vi "Sub Super Duper_6_14b_JW.vi"(0 "VISA resource name":refnum<visa-resource-name>="GPIB0::17::INSTR", 1 "Sample Properties:":T5 {"Date Created" format="%<%Y/%m/%d>T"}, 2 "TRF Cluster":T6={"Step 4"=-38.0, "# of Loops"=1.0, "Transfer 2"=FALSE, "Start 4"=-2.0, "Total Points 2"=2, "Start 3"=40.0, "Stop 2"=-40.0, "Step 3"=-1.0, "Loop Step"=0.0, "Integration Time 3"=0, "Loop Wait"=0.0, "First Step"=0.0} {"Loop Wait" format="%<%H:%M:%S>t"; "Integration Time 3" scale=0.0..2.0; "Step 3" format="%.2f"; "Stop 2" format="%.2f"; "Start 3" format="%.2f"; "Start 4" format="%.2f"; "Step 4" format="%.2f"}, 3 "TSP Cluster":T7={"Transport"=FALSE, "Start 2"=0.0, "Stop 3"=-60.0, "Step 2"=-1.0, "Start"=0.0, "Step"=-10.0, "Total Points"=7, "Integration Time"=0} {"Integration Time" scale=0.0..2.0; "Step" format="%.2f"; "Start" format="%.2f"; "Step 2" format="%.2f"; "Stop 3" format="%.2f"; "Start 2" format="%.2f"}, 4 "Compliance Cluster":T2={"Var1 sweep settings"={"sweep spacing (linear: 0)"=0, "sweep mode"=FALSE, "compliance (V)"=100.0, "compliance (A)"=0.001}, "Var1 sweep settings 2"={"sweep spacing (linear: 0)"=0, "sweep mode"=FALSE, "compliance (V)"=100.0, "compliance (A)"=0.001}, "Var2 step settings 2"={"compliance (A)"=0.001, "compliance (V)"=100.0}, "Var2 step settings"={"compliance (A)"=0.001, "compliance (V)"=100.0}} {"Var2 step settings"."compliance (V)" format="%.2f"; "Var2 step settings"."compliance (A)" format="%^.2e"; "Var2 step settings 2"."compliance (V)" format="%.2f"; "Var2 step settings 2"."compliance (A)" format="%^.2e"; "Var1 sweep settings 2"."compliance (A)" format="%^.2e"; "Var1 sweep settings 2"."compliance (V)" format="%.2f"; "Var1 sweep settings 2"."sweep spacing (linear: 0)" items=["linear", "log 10", "log 25", "log 50"]; "Var1 sweep settings"."compliance (A)" format="%^.2e"; "Var1 sweep settings"."compliance (V)" format="%.2f"; "Var1 sweep settings"."sweep spacing (linear: 0)" items=["linear", "log 10", "log 25", "log 50"]}, 5 "error in":errorcluster, 6 "Saved Folder:":path=path "C:/1DATA/2011", 7 "Wait Cluster":T1 {"Wait Time (s)" format="%.1g"; "Wait Countdown" format="%<%H:%M:%S%1u>t"}, 9 "Stop \nCountdown":bool) -> (8 "Status Indicator":bool, 14 "VISA resource name out":refnum<visa-resource-name>, 15 "TRF Path":path, 16 "TSP Path":path, 17 "Graph Cluster":T3, 18 "Char Cluster":T4, 19 "error out":errorcluster)   [LabVIEW 2011]
uses:
  <vilib>/Platform/TimedLoop/XDataNode/timing_clust.ctl
  <vilib>/Platform/TimedLoop/XDataNode/nitl_modes.ctl
  <vilib>/Platform/TimedLoop/XDataNode/wakeup.ctl
  <vilib>/Platform/TimedLoop/XDataNode/XDataNode.xnode
  <vilib>/Platform/TimedLoop/XDataNode/XDNodeRunTimeDep.lvlib
panel:
  in  "Transport Temp":cluster{"trace":dbl[], "trace":dbl[]}(graph)
  in  "Transfer Temp":cluster{dbl[], "trace":dbl[]}[](graph) caption="Transfer"
  out "graphic display":cluster{"trace":dbl[], "trace":dbl[]}(graph)
  # "Vg Sweep"
  # "Vd Step"
  # "Loops and Integration Time"
  # "Device Characteristics"
  # "Sample Properties:"
  # "%"
  # "nm"
  # "Device Properties:"
  # "um"
  # "um"
  # "Vg Step"
  # "Vd Step"
  # "Integration Time"
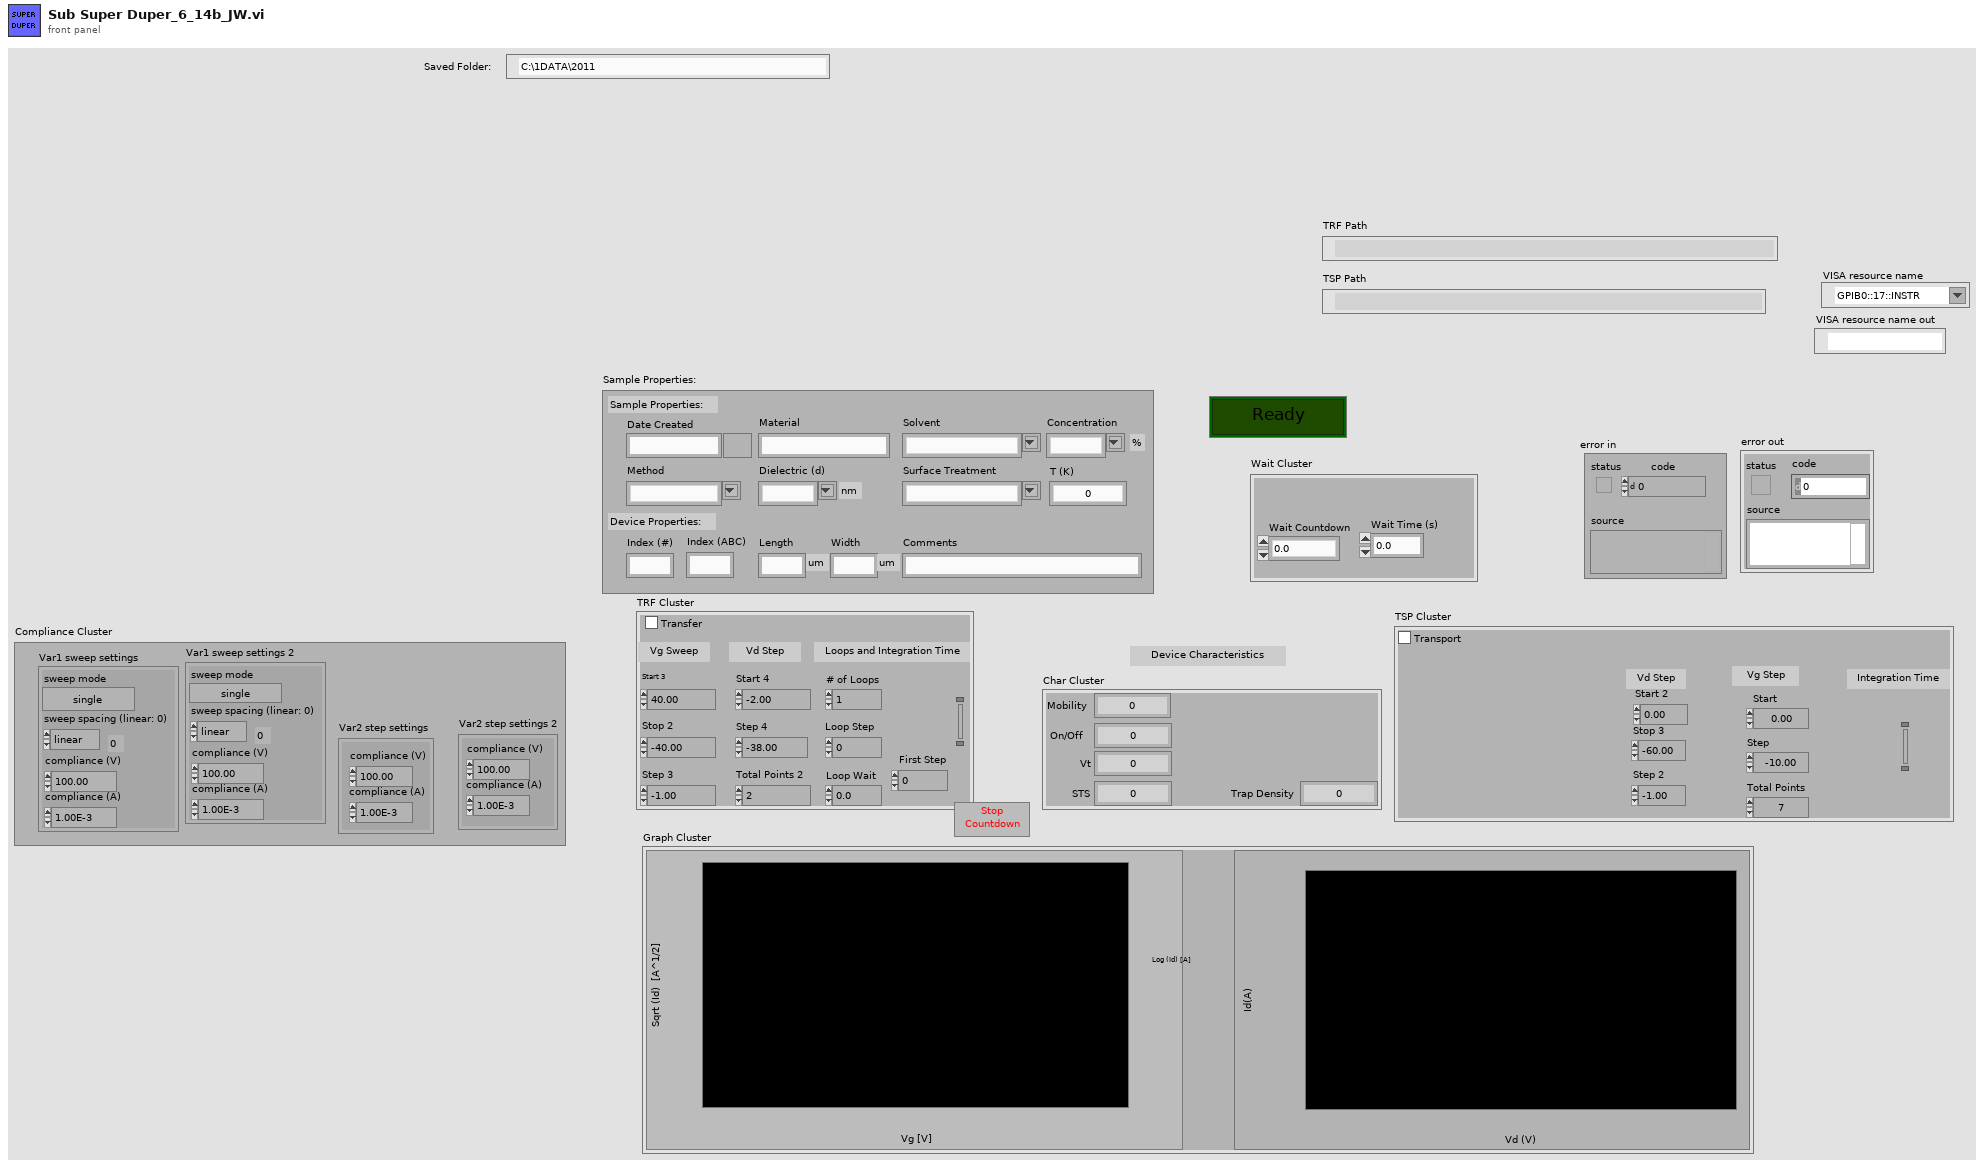
[diagram p1: front panel]
types:
  T1 = cluster{"Wait Countdown":dbl, "Wait Time (s)":dbl}
  T2 = cluster{"Var1 sweep settings":cluster{"sweep spacing (linear: 0)":u16, "sweep mode":bool, "compliance (V)":dbl, "compliance (A)":dbl}, "Var1 sweep settings 2":cluster{"sweep spacing (linear: 0)":u16, "sweep mode":bool, "compliance (V)":dbl, "compliance (A)":dbl}, "Var2 step settings 2":cluster{"compliance (A)":dbl, "compliance (V)":dbl}, "Var2 step settings":cluster{"compliance (A)":dbl, "compliance (V)":dbl}}
  T3 = cluster{"Transfer":cluster{dbl[], "trace":dbl[]}[], "Transport":cluster{"trace":dbl[], "trace":dbl[]}}
  T4 = cluster{"Mobility":dbl, "On/Off ":dbl, "Vt":dbl, "STS":dbl, "Trap Density":dbl}
  T5 = cluster{"Date Created":timestamp, "Material":string, "Solvent":string, "Concentration":string, "Method":string, "Dielectric (d)":string, "Index (#)":string, "Index (ABC)":string, "Length":string, "Width":string, "Surface Treatment":string, "Comments":string, "T (K)":dbl}
  T6 = cluster{"Step 4":dbl, "# of Loops":dbl, "Transfer 2":bool, "Start 4":dbl, "Total Points 2":u16, "Start 3":dbl, "Stop 2":dbl, "Step 3":dbl, "Loop Step":dbl, "Integration Time 3":u32, "Loop Wait":dbl, "First Step":dbl}
  T7 = cluster{"Transport":bool, "Start 2":dbl, "Stop 3":dbl, "Step 2":dbl, "Start":dbl, "Step":dbl, "Total Points":u16, "Integration Time":u32}
  T8 = typedef "XDNodeRunTimeDep.lvlib/timing_clust.ctl" = cluster{"Expected End [f-1]":u64, "Actual End [f-1]":u64, "Finished Late? [f-1]":bool, "Expected End [i-1]":u64, "Actual End [i-1]":u64, "Finished Late? [i-1]":bool, "Expected Start [i]":u64, "Actual Start [i]":u64, "Expected Start [f]":u64, "Actual Start [f]":u64, "Source Name":string, "Structure Name":string, "Period":i64, "Deadline":i64, "Offset":i64, "Start":i64, "Priority":i32, "Timeout":i32, "Mode":T9, "Wakeup Reason":T10, "Error":errorcluster, "Source Type":string, "Secondary Source Type":string, "Global End Time":u64, "Global Start Time":u64, "Frame Duration":u64, "Iteration Duration":u64, "Assigned CPU":i32, "I/O Scan Engine Mode":u32}
  T9 = typedef "XDNodeRunTimeDep.lvlib/nitl_modes.ctl" = enum32{"No Change", "Process missed periods, maintain original phase", "Discard missed periods, maintain original phase", "Process missed periods, ignore original phase", "Discard missed periods, ignore original phase"}
  T10 = typedef "XDNodeRunTimeDep.lvlib/wakeup.ctl" = enum32{"Normal", "Aborted", "Asynchronous wakeup", "Timing source error", "Timed loop error", "Timeout"}
  T11 = cluster{"sweep spacing (linear: 0)":u16, "sweep mode":bool, "compliance (V)":dbl, "compliance (A)":dbl}
  T12 = cluster{"compliance (A)":dbl, "compliance (V)":dbl}
  T13 = cluster{"Start 3":dbl, "Stop 2":dbl, "Step 3":dbl, "sweep spacing (linear: 0)":u16, "sweep mode":bool, "compliance (V)":dbl, "compliance (A)":dbl}
  T14 = cluster{"compliance (A)":dbl, "compliance (V)":dbl, "Start 4":dbl, "Total Points 2":u16, dbl}
  T15 = cluster{"Step 4":dbl, "# of Loops":dbl, "Transfer 2":bool, "Start 4":dbl, "Total Points 2":u16, "Start 3":dbl, "Stop 2":dbl, "Step 3":dbl, dbl, "Integration Time 3":u32, "Loop Wait":dbl, "First Step":dbl}
  T16 = cluster{"Mobility":dbl, "On/Off Current":dbl, "Vt":dbl, "Trap Density":dbl, "STS":dbl}
  T17 = cluster{"Start 2":dbl, "Stop 3":dbl, "Step 2":dbl, "sweep spacing (linear: 0)":u16, "sweep mode":bool, "compliance (V)":dbl, "compliance (A)":dbl}
  T18 = cluster{"compliance (A)":dbl, "compliance (V)":dbl, "Start":dbl, "Total Points":u16, "Step":dbl}
  T19 = cluster{"Transfer Temp":cluster{dbl[], "trace":dbl[]}[], "Transport Temp":cluster{"trace":dbl[], "trace":dbl[]}}
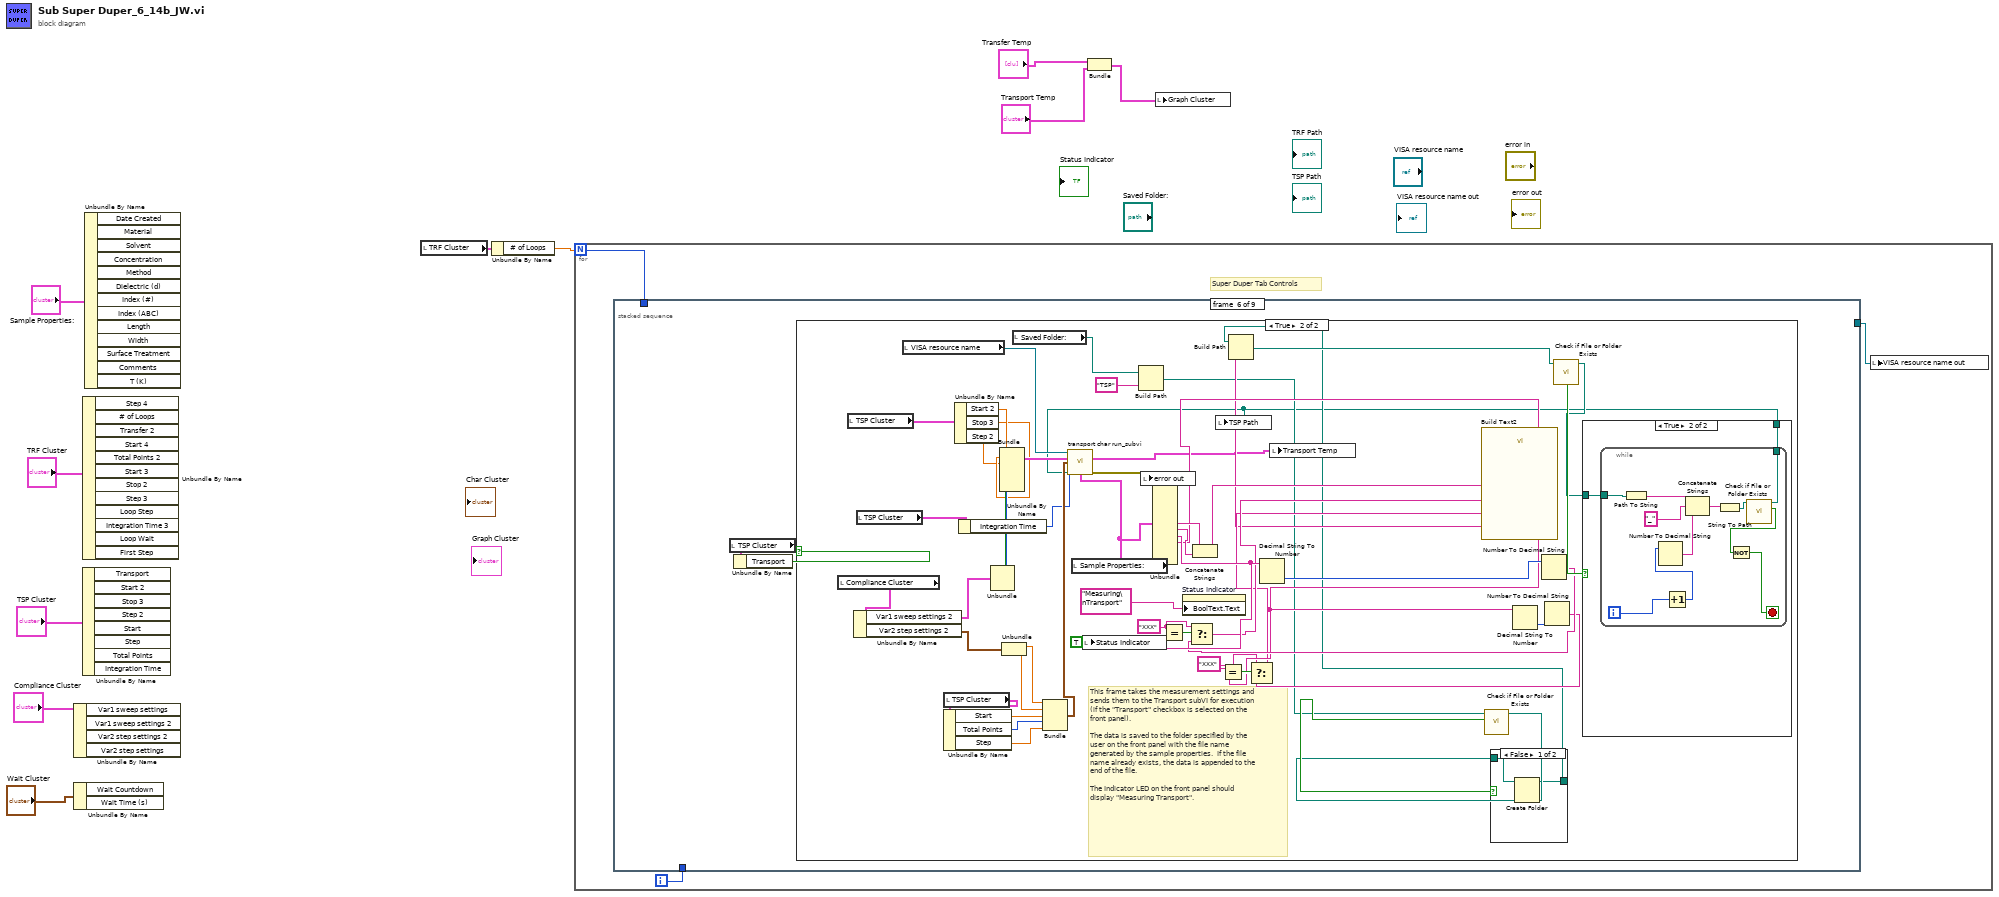
[diagram p0: block diagram]
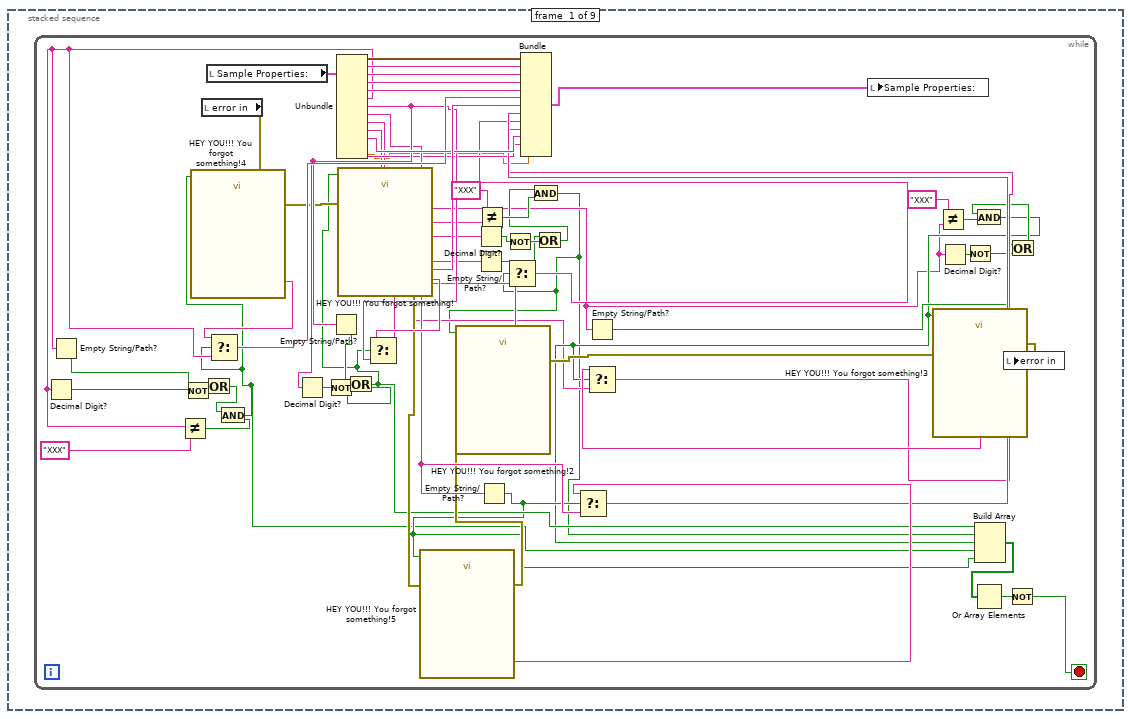
[diagram p2: hidden frame]
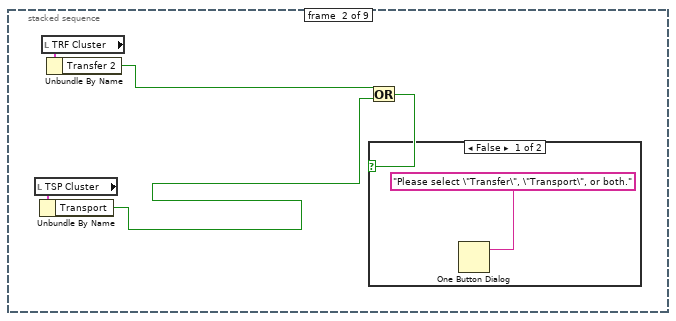
[diagram p3: hidden frame]
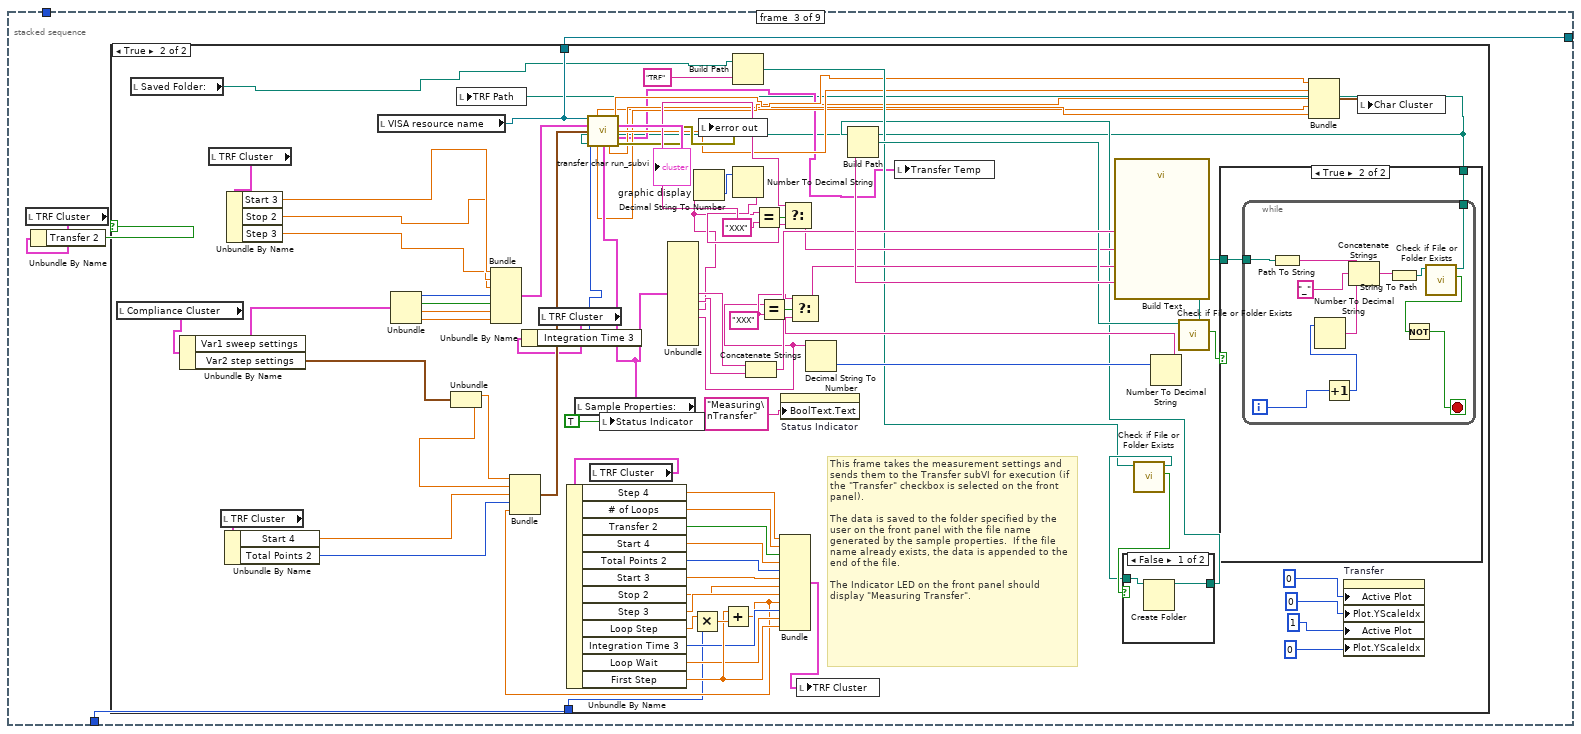
[diagram p5: hidden frame]
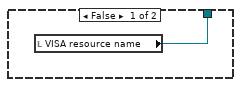
[diagram p6: hidden frame]
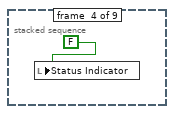
[diagram p9: hidden frame]
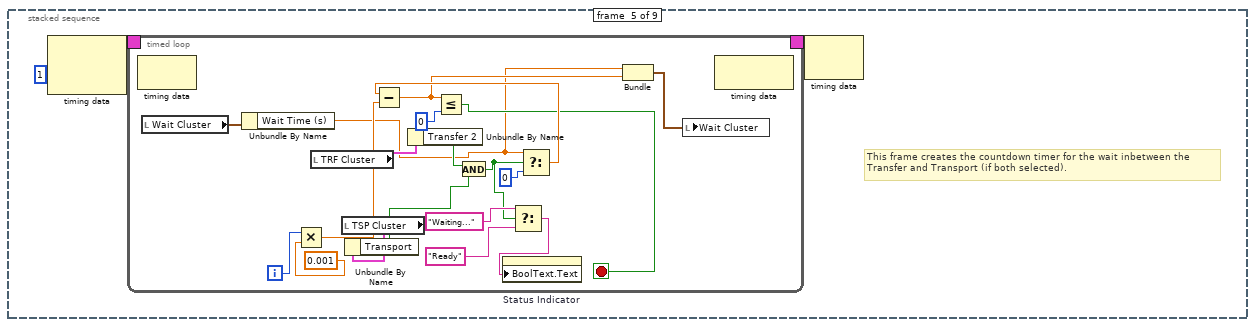
[diagram p10: hidden frame]
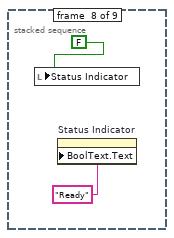
[diagram p15: hidden frame]
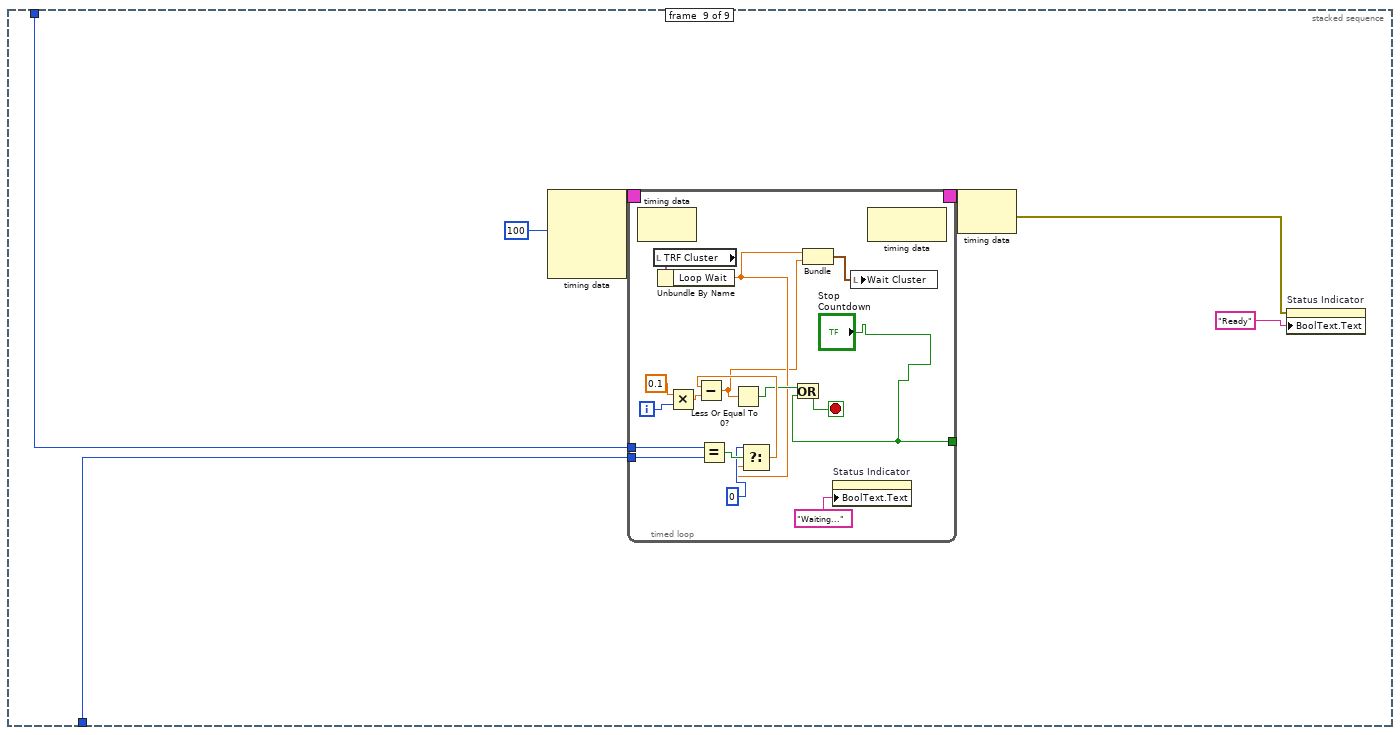
[diagram p16: hidden frame]
diagram:
  n1 = Unbundle By Name("Compliance Cluster") -> ()  [unwired: 4 out]
  n2 = Unbundle By Name("Wait Cluster") -> ()  [unwired: 2 out]
  n3 = Unbundle By Name("TSP Cluster") -> ()  [unwired: 8 out]
  n4 = Unbundle By Name("TRF Cluster") -> ()  [unwired: 12 out]
  n5 = Unbundle By Name("Sample Properties:") -> ()  [unwired: 13 out]
  n6 = local read "TRF Cluster"() -> (w10:T6)
  n7 = Unbundle By Name(w10) -> ("# of Loops"=w9:dbl)
  n8 = for {
    N: w9 -> [w12]
    i -> [w13]
    # "Super Duper Tab Controls"
    n9 = stacked-sequence {
      tunnel: w13 -> [_ _ w83 _ _ _ _ _ w286]
      tunnel: w12 -> [_ _ _ _ _ _ _ _ w285]
      tunnel: [_ _ w80 _ _ _ _ _ _] -> w11
      frame #0 {
        n10 = while {
          stop <- w39 stop-if-true
          n11 = local read "error in"() -> (w45:errorcluster)
          n12 = local read "Sample Properties:"() -> (w68:T5)
          n13 = Unbundle(w68) -> ("Date Created"=w69:timestamp, "Material"=w70:string, "Solvent"=w71:string, "Concentration"=w72:string, "Method"=w73:string, "Dielectric (d)"=w28:string, "Index (#)"=w58:string, "Index (ABC)"=w55:string, "Length"=w23:string, "Width"=w16:string, "Surface Treatment"=w61:string, "Comments"=w53:string, "T (K)"=w14:dbl)
          n14 = Decimal Digit?(1:w28) -> (0:w36:bool)
          n15 = Empty String/Path?(string/path=w28) -> (empty?=w30:bool)
          n16 = Not Equal?(x=w28, y="XXX") -> (x != y?=w27:bool)
          n17 = Not(x=w36) -> (.not. x?=w33:bool)
          n18 = Or(x=w30, y=w33) -> (x .or. y?=w26:bool)
          n19 = And(x=w26, y=w27) -> (x .and. y?=w25:bool)
          n20 = call "HEY YOU!!! You forgot something!4"("Enable"=w25, "error in (no error)"=w45) -> ("Dielectric (d)"=w60:string, "error out"=w44:errorcluster)  [unwired: 15 in, 1 out]
          n21 = Select(t=w60, s=w25, f=w28) -> (s? t:f=w59:string)
          n22 = Decimal Digit?(1:w58) -> (0:w49:bool)
          n23 = Not(x=w49) -> (.not. x?=w48:bool)
          n24 = Empty String/Path?(string/path=w58) -> (empty?=w57:bool)
          n25 = Or(x=w57, y=w48) -> (x .or. y?=w43:bool)
          n26 = call "HEY YOU!!! You forgot something!"("Enable"=w43, "error in (no error)"=w44) -> ("Index (#)"=w67:string, "error out"=w47:errorcluster)  [unwired: 15 in, 1 out]
          n27 = Select(t=w67, s=w43, f=w58) -> (s? t:f=w64:string)
          n28 = Decimal Digit?(1:w23) -> (0:w38:bool)
          n29 = Empty String/Path?(string/path=w23) -> (empty?=w32:bool)
          n30 = Not Equal?(x="XXX", y=w23) -> (x != y?=w22:bool)
          n31 = Empty String/Path?(string/path=w55) -> (empty?=w42:bool)
          n32 = call "HEY YOU!!! You forgot something!5"("Enable"=w42, "error in (no error)"=w47) -> ("Index (ABC)"=w56:string, "error out"=w46:errorcluster)  [unwired: 15 in, 1 out]
          n33 = Not(x=w38) -> (.not. x?=w35:bool)
          n34 = Or(x=w32, y=w35) -> (x .or. y?=w21:bool)
          n35 = And(x=w21, y=w22) -> (x .and. y?=w15:bool)
          n36 = call "HEY YOU!!! You forgot something!2"("Enable"=w15, "error in (no error)"=w46) -> ("Length"=w66:string, "error out"=w63:errorcluster)  [unwired: 15 in, 1 out]
          n37 = Select(t=w66, s=w15, f=w23) -> (s? t:f=w52:string)
          n38 = Select(t=w56, s=w42, f=w55) -> (s? t:f=w54:string)
          n39 = Empty String/Path?(string/path=w16) -> (empty?=w31:bool)
          n40 = Not Equal?(x="XXX", y=w16) -> (x != y?=w20:bool)
          n41 = Decimal Digit?(1:w16) -> (0:w37:bool)
          n42 = Not(x=w37) -> (.not. x?=w34:bool)
          n43 = Or(x=w31, y=w34) -> (x .or. y?=w19:bool)
          n44 = And(x=w19, y=w20) -> (x .and. y?=w18:bool)
          n45 = call "HEY YOU!!! You forgot something!3"("Enable"=w18, "error in (no error)"=w63) -> ("Width"=w65:string, "error out"=w62:errorcluster)  [unwired: 15 in, 1 out]
          n46 = Select(t=w65, s=w18, f=w16) -> (s? t:f=w51:string)
          n47 = Bundle("Date Created"=w69, "Material"=w70, "Solvent"=w71, "Concentration"=w72, "Method"=w73, "Dielectric (d)"=w59, "Index (#)"=w64, "Index (ABC)"=w54, "Length"=w52, "Width"=w51, "Surface Treatment"=w61, "Comments"=w53, "T (K)"=w14) -> (w50:T5)  [unwired: 1 in]
          n48 = local write "Sample Properties:"(w50) -> ()
          n49 = Build Array(w43, w15, w18, w25, w42) -> (w41:bool[])
          n50 = Or Array Elements(Boolean array=w41) -> (logical OR=w40:bool)
          n51 = local write "error in"(w62) -> ()
          n52 = Not(x=w40) -> (.not. x?=w39:bool)
        }
      }
      frame #1 {
        n53 = local read "TSP Cluster"() -> (w75:T7)
        n54 = Unbundle By Name(w75) -> ("Transport"=w74:bool)
        n55 = local read "TRF Cluster"() -> (w77:T6)
        n56 = Unbundle By Name(w77) -> ("Transfer 2"=w76:bool)
        n57 = Or(x=w76, y=w74) -> (x .or. y?=w78:bool)
        n58 = case shown="False" w78 {
          frame False {
            n59 = One Button Dialog(message="Please select \"Transfer\", \"Transport\", or both.") -> ()  [unwired: 1 in, 1 out]
          }
          frame True {
          }
        }
      }
      frame #2 {
        n60 = local read "TRF Cluster"() -> (w81:T6)
        n61 = Unbundle By Name(w81) -> ("Transfer 2"=w82:bool)
        n62 = case shown="True" w82 {
          tunnel: w83 -> [_ w98]
          tunnel: [w84 w90] -> w80
          frame False {
            n63 = local read "VISA resource name"() -> (w84:refnum<visa-resource-name>)
          }
          frame True {
            w139 = "XXX"
            w143 = "XXX"
            # "This frame takes the measurement settings and sends them to the Transfer subVI for execution (if the \"Transfer\" checkbox is selected on the front panel).\n\nThe data is saved to the folder specified by the user on the front panel with the file name generated by the sample properties.  If the file name already exists, the data is appended to the end of the file.\n\nThe Indicator LED on the front panel should display \"Measuring Transfer\"."
            n64 = local read "Compliance Cluster"() -> (w87:T2)
            n65 = local read "Saved Folder:"() -> (w89:path)
            n66 = Unbundle By Name(w87) -> ("Var1 sweep settings"=w85:T11, "Var2 step settings"=w86:T12)
            n67 = local read "TRF Cluster"() -> (w120:T6)
            n68 = local read "TRF Cluster"() -> (w123:T6)
            n69 = Unbundle By Name(w123) -> ("Start 4"=w122:dbl, "Total Points 2"=w121:u16)
            n70 = Unbundle By Name(w120) -> ("Start 3"=w119:dbl, "Stop 2"=w118:dbl, "Step 3"=w117:dbl)
            n71 = local read "VISA resource name"() -> (w90:refnum<visa-resource-name>)
            n72 = Unbundle(w85) -> ("sweep spacing (linear: 0)"=w164:u16, "sweep mode"=w163:bool, "compliance (V)"=w162:dbl, "compliance (A)"=w161:dbl)
            n73 = Unbundle(w86) -> ("compliance (A)"=w159:dbl, "compliance (V)"=w158:dbl)
            n74 = Bundle("Start 3"=w119, "Stop 2"=w118, "Step 3"=w117, "sweep spacing (linear: 0)"=w164, "sweep mode"=w163, "compliance (V)"=w162, "compliance (A)"=w161) -> (w160:T13)  [unwired: 1 in]
            n75 = local read "TRF Cluster"() -> (w115:T6)
            n76 = Unbundle By Name(w115) -> ("Integration Time 3"=w116:u32)
            n77 = local read "Sample Properties:"() -> (w125:T5)
            n78 = local read "TRF Cluster"() -> (w101:T6)
            n79 = Unbundle By Name(w101) -> ("Step 4"=w102:dbl, "# of Loops"=w103:dbl, "Transfer 2"=w104:bool, "Start 4"=w105:dbl, "Total Points 2"=w106:u16, "Start 3"=w107:dbl, "Stop 2"=w108:dbl, "Step 3"=w109:dbl, "Loop Step"=w112:dbl, "Integration Time 3"=w110:u32, "Loop Wait"=w111:dbl, "First Step"=w113:dbl)
            n80 = local write "Status Indicator"(TRUE) -> ()
            n81 = Unbundle(w125) -> ("Index (#)"=w152:string, "Index (ABC)"=w151:string, "Length"=w135:string, "Width"=w138:string)  [unwired: 9 out]
            n82 = Multiply(x=w112, y=w98) -> (x*y=w114:dbl)
            n83 = Decimal String To Number(string=w135) -> (number=w146:i32)  [unwired: 2 in, 1 out]
            n84 = Add(x=w113, y=w114) -> (x+y=w100:dbl)
            n85 = Bundle("compliance (A)"=w159, "compliance (V)"=w158, "Start 4"=w122, "Total Points 2"=w121, w100) -> (w157:T14)  [unwired: 1 in]
            n86 = Build Path(base path=w89, name or relative path="TRF") -> (appended path=w131:path)
            n87 = Number To Decimal String(number=w146) -> (decimal integer string=w142:string)  [unwired: 1 in]
            n88 = Concatenate Strings(w152, w151) -> (w150:string)
            n89 = Equal?(x=w135, y=w143) -> (x = y?=w144:bool)
            n90 = Equal?(x=w138, y=w139) -> (x = y?=w140:bool)
            n91 = Bundle ("Bundle Again")("Step 4"=w102, "# of Loops"=w103, "Transfer 2"=w104, "Start 4"=w105, "Total Points 2"=w106, "Start 3"=w107, "Stop 2"=w108, "Step 3"=w109, w100, "Integration Time 3"=w110, "Loop Wait"=w111, "First Step"=w113) -> (w99:T15)  [unwired: 1 in]
            n92 = property on="Status Indicator" class="Bool (strict)"("BoolText.Text"="Measuring\nTransfer") -> ()  [unwired: 2 in, 2 out]
            n93 = Select(t=w143, s=w144, f=w142) -> (s? t:f=w141:string)
            n94 = local write "TRF Cluster"(w99) -> ()
            n95 = Decimal String To Number(string=w138) -> (number=w145:i32)  [unwired: 2 in, 1 out]
            n96 = call <vilib>:"Check if File or Folder Exists.vi"("path"=w131) -> ("file or folder exists?"=w133:bool, "dup path"=w132:path)  [unwired: 8 in, 1 out]
            n97 = case shown="False" w133 {
              tunnel: w132 -> [w166 w167]
              tunnel: [w165 w167] -> w130
              frame False {
                n98 = Create Folder(path (use dialog)=w166) -> (created path=w165:path)  [unwired: 2 in, 2 out]
              }
              frame True {
              }
            }
            n99 = Number To Decimal String(number=w145) -> (decimal integer string=w137:string)  [unwired: 1 in]
            n100 = Select(t=w139, s=w140, f=w137) -> (s? t:f=w136:string)
            n101 = call "Build Text"("Index"=w150, "Length"=w141, "Width"=w136) -> ("Result"=w156:string)  [unwired: 11 in, 1 out]
            n102 = Build Path(base path=w130, name or relative path=w156) -> (appended path=w148:path)
            n103 = call <vilib>:"Check if File or Folder Exists.vi"("path"=w148) -> ("file or folder exists?"=w149:bool, "dup path"=w147:path)  [unwired: 8 in, 1 out]
            n104 = case shown="True" w149 {
              tunnel: w147 -> [w168 w170]
              tunnel: [w168 w169] -> w88
              frame False {
              }
              frame True {
                n105 = while {
                  tunnel: w170 -> [w172]
                  tunnel: [w171] -> w169
                  i -> [w174]
                  stop <- w175 stop-if-true
                  n106 = Path To String(path=w172) -> (string=w181:string)
                  n107 = Increment(x=w174) -> (x+1=w173:i32)
                  n108 = Number To Decimal String(number=w173) -> (decimal integer string=w179:string)  [unwired: 1 in]
                  n109 = Concatenate Strings(w181, "_", w179) -> (w178:string)
                  n110 = String To Path(string=w178) -> (path=w177:path)
                  n111 = call <vilib>:"Check if File or Folder Exists.vi"("path"=w177) -> ("file or folder exists?"=w176:bool, "dup path"=w171:path)  [unwired: 8 in, 1 out]
                  n112 = Not(x=w176) -> (.not. x?=w175:bool)
                }
              }
            }
            n113 = local write "TRF Path"(w88) -> ()
            n114 = call "transfer char run_subvi.vi"("VISA session"=w90, "Var1 sweep settings"=w160, "Var2 step settings"=w157, "integration time"=w116, "Path"=w88, "Sample Properties:"=w125) -> ("Trap Density"=w92:dbl, "Mobility"=w96:dbl, "graphic display"=→"graphic display":cluster{"trace":dbl[], "trace":dbl[]}, "On/Off Current"=w95:dbl, "XY Graph"=w91:cluster{dbl[], "trace":dbl[]}[], "Vt"=w94:dbl, "STS"=w93:dbl, "error?"=w124:errorcluster)  [unwired: 2 in]
            n115 = local write "error out"(w124) -> ()
            n116 = local write "Transfer Temp"(w91) -> ()
            n117 = Bundle("Mobility"=w96, "On/Off Current"=w95, "Vt"=w94, "Trap Density"=w92, "STS"=w93) -> (w97:T16)  [unwired: 1 in]
            n118 = property on="Transfer" class="XYGraph (strict)"("Active Plot"=0, "Plot.YScaleIdx"=0, "Active Plot"=1, "Plot.YScaleIdx"=0) -> ()  [unwired: 2 in, 2 out]
            n119 = local write "Char Cluster"(w97) -> ()
          }
        }
      }
      frame #3 {
        n120 = local write "Status Indicator"(FALSE) -> ()
      }
      frame #4 {
        # "This frame creates the countdown timer for the wait inbetween the\nTransfer and Transport (if both selected)."
        n121 = node-c288(1) -> (w185:T8)  [unwired: 1 in]
        n122 = timed-loop {
          timing: w185 -> [_]
          timing-out: [_] -> w184
          i -> [w196]
          stop <- w197 stop-if-true
          n123 = node-c288() -> ()  [unwired: 1 in, 1 out]
          n124 = local read "Wait Cluster"() -> (w189:T1)
          n125 = Unbundle By Name(w189) -> ("Wait Time (s)"=w187:dbl)
          n126 = Multiply(x=w196, y=0.001) -> (x*y=w194:dbl)
          n127 = local read "TRF Cluster"() -> (w190:T6)
          n128 = local read "TSP Cluster"() -> (w191:T7)
          n129 = Unbundle By Name(w191) -> ("Transport"=w192:bool)
          n130 = Unbundle By Name(w190) -> ("Transfer 2"=w193:bool)
          n131 = And(x=w193, y=w192) -> (x .and. y?=w201:bool)
          n132 = Select(t="Waiting...", s=w201, f="Ready") -> (s? t:f=w203:string)
          n133 = property on="Status Indicator" class="Bool (strict)"("BoolText.Text"=w203) -> ()  [unwired: 2 in, 2 out]
          n134 = Select(t=w187, s=w201, f=0) -> (s? t:f=w199:dbl)
          n135 = Subtract(x=w199, y=w194) -> (x-y=w188:dbl)
          n136 = Less Or Equal?(x=w188, y=0) -> (x <= y?=w197:bool)
          n137 = Bundle("Wait Time (s)"=w187, w188) -> (w186:cluster{"Wait Time (s)":dbl, dbl})  [unwired: 1 in]
          n138 = local write "Wait Cluster"(w186) -> ()
          n139 = node-c288() -> ()  [unwired: 1 in, 1 out]
        }
        n140 = node-c288(w184) -> ()  [unwired: 1 out]
      }
      frame #5 {
        n141 = local read "TSP Cluster"() -> (w212:T7)
        n142 = Unbundle By Name(w212) -> ("Transport"=w211:bool)
        n143 = case shown="True" w211 {
          frame False {
          }
          frame True {
            w238 = "XXX"
            w242 = "XXX"
            # "This frame takes the measurement settings and sends them to the Transport subVI for execution (if the \"Transport\" checkbox is selected on the front panel).\n\nThe data is saved to the folder specified by the user on the front panel with the file name generated by the sample properties.  If the file name already exists, the data is appended to the end of the file.\n\nThe Indicator LED on the front panel should display \"Measuring Transport\"."
            n144 = local read "Compliance Cluster"() -> (w216:T2)
            n145 = local read "TSP Cluster"() -> (w229:T7)
            n146 = Unbundle By Name(w216) -> ("Var1 sweep settings 2"=w215:T11, "Var2 step settings 2"=w214:T12)
            n147 = local read "TSP Cluster"() -> (w222:T7)
            n148 = local read "VISA resource name"() -> (w218:refnum<visa-resource-name>)
            n149 = local read "TSP Cluster"() -> (w220:T7)
            n150 = Unbundle By Name(w220) -> ("Start"=w225:dbl, "Total Points"=w224:u16, "Step"=w223:dbl)
            n151 = Unbundle By Name(w229) -> ("Start 2"=w228:dbl, "Stop 3"=w227:dbl, "Step 2"=w226:dbl)
            n152 = Unbundle By Name(w222) -> ("Integration Time"=w221:u32)
            n153 = Unbundle(w215) -> ("sweep spacing (linear: 0)"=w265:u16, "sweep mode"=w264:bool, "compliance (V)"=w263:dbl, "compliance (A)"=w262:dbl)
            n154 = Bundle("Start 2"=w228, "Stop 3"=w227, "Step 2"=w226, "sweep spacing (linear: 0)"=w265, "sweep mode"=w264, "compliance (V)"=w263, "compliance (A)"=w262) -> (w261:T17)  [unwired: 1 in]
            n155 = Unbundle(w214) -> ("compliance (A)"=w260:dbl, "compliance (V)"=w259:dbl)
            n156 = local read "Saved Folder:"() -> (w217:path)
            n157 = Bundle("compliance (A)"=w260, "compliance (V)"=w259, "Start"=w225, "Total Points"=w224, "Step"=w223) -> (w258:T18)  [unwired: 1 in]
            n158 = local read "Sample Properties:"() -> (w254:T5)
            n159 = local write "Status Indicator"(TRUE) -> ()
            n160 = Build Path(base path=w217, name or relative path="TSP") -> (appended path=w231:path)
            n161 = Unbundle(w254) -> ("Index (#)"=w253:string, "Index (ABC)"=w252:string, "Length"=w243:string, "Width"=w239:string)  [unwired: 9 out]
            n162 = Equal?(x=w242, y=w243) -> (x = y?=w244:bool)
            n163 = property on="Status Indicator" class="Bool (strict)"("BoolText.Text"="Measuring\nTransport") -> ()  [unwired: 2 in, 2 out]
            n164 = Concatenate Strings(w253, w252) -> (w251:string)
            n165 = Equal?(x=w238, y=w239) -> (x = y?=w247:bool)
            n166 = Decimal String To Number(string=w243) -> (number=w246:i32)  [unwired: 2 in, 1 out]
            n167 = call <vilib>:"Check if File or Folder Exists.vi"("path"=w231) -> ("file or folder exists?"=w233:bool, "dup path"=w232:path)  [unwired: 8 in, 1 out]
            n168 = case shown="False" w233 {
              tunnel: w232 -> [w267 w268]
              tunnel: [w266 w268] -> w230
              frame False {
                n169 = Create Folder(path (use dialog)=w267) -> (created path=w266:path)  [unwired: 2 in, 2 out]
              }
              frame True {
              }
            }
            n170 = Decimal String To Number(string=w239) -> (number=w245:i32)  [unwired: 2 in, 1 out]
            n171 = Number To Decimal String(number=w246) -> (decimal integer string=w241:string)  [unwired: 1 in]
            n172 = Select(t=w242, s=w244, f=w241) -> (s? t:f=w240:string)
            n173 = Number To Decimal String(number=w245) -> (decimal integer string=w237:string)  [unwired: 1 in]
            n174 = Select(t=w238, s=w247, f=w237) -> (s? t:f=w236:string)
            n175 = call "Build Text2"("Index"=w251, "Length"=w240, "Width"=w236) -> ("Result"=w235:string)  [unwired: 11 in, 1 out]
            n176 = Build Path(base path=w230, name or relative path=w235) -> (appended path=w248:path)
            n177 = call <vilib>:"Check if File or Folder Exists.vi"("path"=w248) -> ("file or folder exists?"=w250:bool, "dup path"=w249:path)  [unwired: 8 in, 1 out]
            n178 = case shown="True" w250 {
              tunnel: w249 -> [w269 w271]
              tunnel: [w269 w270] -> w213
              frame False {
              }
              frame True {
                n179 = while {
                  tunnel: w271 -> [w273]
                  tunnel: [w272] -> w270
                  i -> [w275]
                  stop <- w276 stop-if-true
                  n180 = Path To String(path=w273) -> (string=w282:string)
                  n181 = Increment(x=w275) -> (x+1=w274:i32)
                  n182 = Number To Decimal String(number=w274) -> (decimal integer string=w280:string)  [unwired: 1 in]
                  n183 = Concatenate Strings(w282, "_", w280) -> (w279:string)
                  n184 = String To Path(string=w279) -> (path=w278:path)
                  n185 = call <vilib>:"Check if File or Folder Exists.vi"("path"=w278) -> ("file or folder exists?"=w277:bool, "dup path"=w272:path)  [unwired: 8 in, 1 out]
                  n186 = Not(x=w277) -> (.not. x?=w276:bool)
                }
              }
            }
            n187 = call "transport char run_subvi.vi"("VISA session"=w218, "Var1 sweep settings"=w261, "Var2 step settings"=w258, "integration time"=w221, "Path"=w213, "Sample Properties:"=w254) -> ("graphic display"=w219:cluster{"trace":dbl[], "trace":dbl[]}, "error?"=w257:errorcluster)  [unwired: 8 in]
            n188 = local write "error out"(w257) -> ()
            n189 = local write "TSP Path"(w213) -> ()
            n190 = local write "Transport Temp"(w219) -> ()
          }
        }
      }
      frame #6 {
      }
      frame #7 {
        n191 = local write "Status Indicator"(FALSE) -> ()
        n192 = property on="Status Indicator" class="Bool (strict)"("BoolText.Text"="Ready") -> ()  [unwired: 2 in, 2 out]
      }
      frame #8 {
        n193 = node-c288(100) -> (w291:T8)  [unwired: 3 in]
        n194 = timed-loop {
          timing: w291 -> [_]
          timing-out: [_] -> w290
          tunnel: w286 -> [w302]
          tunnel: w285 -> [w301]
          tunnel: ["Stop \nCountdown"] -> _
          i -> [w307]
          stop <- w297 stop-if-true
          n195 = node-c288() -> ()  [unwired: 1 in, 1 out]
          n196 = local read "TRF Cluster"() -> (w296:T6)
          n197 = Unbundle By Name(w296) -> ("Loop Wait"=w294:dbl)
          n198 = Multiply(x=0.1, y=w307) -> (x*y=w305:dbl)
          n199 = Equal?(x=w301, y=w302) -> (x = y?=w303:bool)
          n200 = Select(t=0, s=w303, f=w294) -> (s? t:f=w299:dbl)
          n201 = Subtract(x=w299, y=w305) -> (x-y=w293:dbl)
          n202 = Less Or Equal To 0?(x=w293) -> (x <= 0?=w298:bool)
          n203 = Or(x=w298, y="Stop \nCountdown") -> (x .or. y?=w297:bool)
          n204 = Bundle("Loop Wait"=w294, w293) -> (w295:cluster{"Loop Wait":dbl, dbl})  [unwired: 1 in]
          n205 = property on="Status Indicator" class="Bool (strict)"("BoolText.Text"="Waiting...") -> ()  [unwired: 2 in, 2 out]
          n206 = local write "Wait Cluster"(w295) -> ()
          n207 = node-c288() -> ()  [unwired: 1 in, 1 out]
        }
        n208 = node-c288(w290) -> (w287:errorcluster)
        n209 = property on="Status Indicator" class="Bool (strict)"(error in=w287, "BoolText.Text"="Ready") -> ()  [unwired: 1 in, 2 out]
      }
    }
    n210 = local write "VISA resource name out"(w11) -> ()
  }
  n211 = Bundle("Transfer Temp"="Transfer Temp", "Transport Temp"="Transport Temp") -> (w6:T19)  [unwired: 1 in]
  n212 = local write "Graph Cluster"(w6) -> ()
